vi "PD Control.vi"(8 "First Run?":bool, 9 "kD":dbl, 10 "kP":dbl, 11 "Error":dbl) -> (2 "PD":dbl)   [LabVIEW 2017]
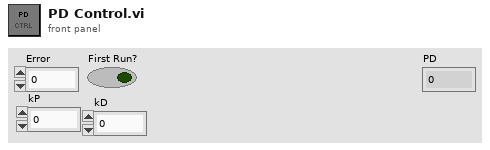
[diagram p1: front panel]
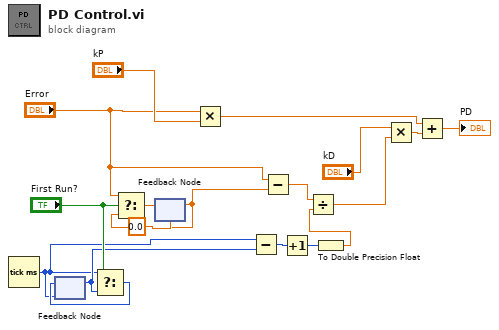
[diagram p0: block diagram]
diagram:
  n1 = Tick Count (ms)() -> (millisecond timer value=w9:u32)
  n2 = feedback #1(w9) -> (w10:u32)
  n3 = Select(t=w9, s="First Run?", f=w10) -> (s? t:f=w13:u32)
  n4 = feedback-in #1(w13) -> ()
  n5 = feedback #2(0.0 ("Error")) -> (w12:dbl)
  n6 = Select(t="Error", s="First Run?", f=w12) -> (s? t:f=w16:dbl)
  n7 = feedback-in #2(w16) -> ()
  n8 = Multiply(x="Error", y="kP") -> (x*y=w17:dbl)
  n9 = Subtract(x=w9, y=w10) -> (x-y=w7:u32)
  n10 = Subtract(x="Error", y=w12) -> (x-y=w8:dbl)
  n11 = Increment(x=w7) -> (x+1=w6:u32)
  n12 = To Double Precision Float(number=w6) -> (double precision float=w5:dbl)
  n13 = Divide(x=w8, y=w5) -> (x/y=w3:dbl)
  n14 = Multiply(x="kD", y=w3) -> (x*y=w2:dbl)
  n15 = Add(x=w17, y=w2) -> (x+y=→"PD":dbl)
